vi "Generate SQL Values.vi"(8 "error in (no error)":errorcluster, 11 "Credit Record in":refnum<class "Credit Transaction.lvclass">) -> (0 "error out":errorcluster, 2 "SQL Values":string, 3 "Credit Record out":refnum<class "Credit Transaction.lvclass">)   [LabVIEW 2018, in "Credit Transaction.lvclass"]
uses:
  Credit Transaction.lvclass
  Credit Transaction.lvclass/Credit Transaction.ctl
  Transaction/Transaction.lvclass
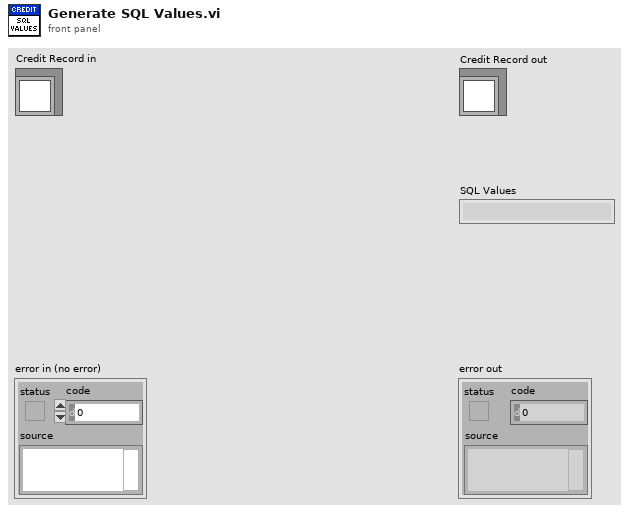
[diagram p1: front panel]
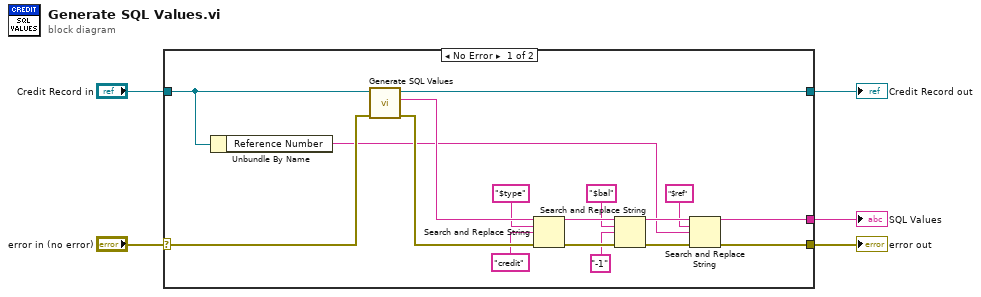
[diagram p0: block diagram]
diagram:
  n1 = case shown="No Error" "error in (no error)" {
    selector: "error in (no error)" -> [w22 w24]
    tunnel: [w15 w24] -> w2
    tunnel: [w12 _] -> w1
    tunnel: "Credit Record in" -> [w9 w23]
    tunnel: [w8 w23] -> w3
    frame No Error {
      n2 = Unbundle By Name(w9) -> ("Reference Number"=w6:string)
      n3 = call-parent "Generate SQL Values.vi"("error in (no error)"=w22, "Transaction in"=w9) -> ("error out"=w21:errorcluster, "SQL Values"=w20:string, "Transaction out"=w8:refnum<class "Credit Transaction.lvclass">)  [unwired: 7 in]
      n4 = Search and Replace String(input string=w20, search string="$type", replace string="credit" ("replace string (\"\")"), error in=w21) -> (result string=w14:string, error out=w17:errorcluster)  [unwired: 4 in, 2 out]
      n5 = Search and Replace String(input string=w14, search string="$bal", replace string="-1" ("replace string (\"\")"), error in=w17) -> (result string=w13:string, error out=w16:errorcluster)  [unwired: 4 in, 2 out]
      n6 = Search and Replace String(input string=w13, search string="$ref", replace string=w6, error in=w16) -> (result string=w12:string, error out=w15:errorcluster)  [unwired: 4 in, 2 out]
    }
    frame Error {
    }
  }
  "error out" <- w2
  "Credit Record out" <- w3
  "SQL Values" <- w1
